vi "Aim Robot.vi"(10 "Drive Speed":dbl, 11 "RobotDriveDevRef":T1={"DevStatus"={"status"=FALSE, "code"=0, "source"=""}, "Motors[]"=[], "Square Inputs"=FALSE, "Max Output"=1.0}) -> (0 "Error Out":string, 3 "RobotDriveDevRef Out":T1={"DevStatus"={"status"=FALSE, "code"=0, "source"=""}, "Motors[]"=[], "Square Inputs"=FALSE, "Max Output"=1.0})   [LabVIEW 2016]
uses:
  <vilib>/Rock Robotics/WPI/RobotDrive/WPI_RobotDriveDevRef.ctl
  <vilib>/Rock Robotics/WPI/MotorControl/WPI_MotorControlDeviceRef.ctl
  <vilib>/Rock Robotics/WPI/MotorControl/WPI_MotorControlType.ctl
  <vilib>/Rock Robotics/SystemInterfaces/DIO/FPGA_DIOPWMChannel.ctl
  <vilib>/Rock Robotics/WPI/PWM/WPI_PWMDeadband.ctl
  <vilib>/Rock Robotics/WPI/Relay/WPI_RelayValue.ctl
  Robot Global Data.vi
  <vilib>/Rock Robotics/Network Tables/NT Read Boolean.vi
  <vilib>/Rock Robotics/WPI/RobotDrive/WPI_RobotDriveArcadeDrive_Standard(NoSaturation).vi
  <vilib>/Rock Robotics/Network Tables/NT Write Numeric Array.vi
  <vilib>/Rock Robotics/Network Tables/NT Read Number.vi
panel:
  out "Drive Motor Values":dbl[](array[numeric])
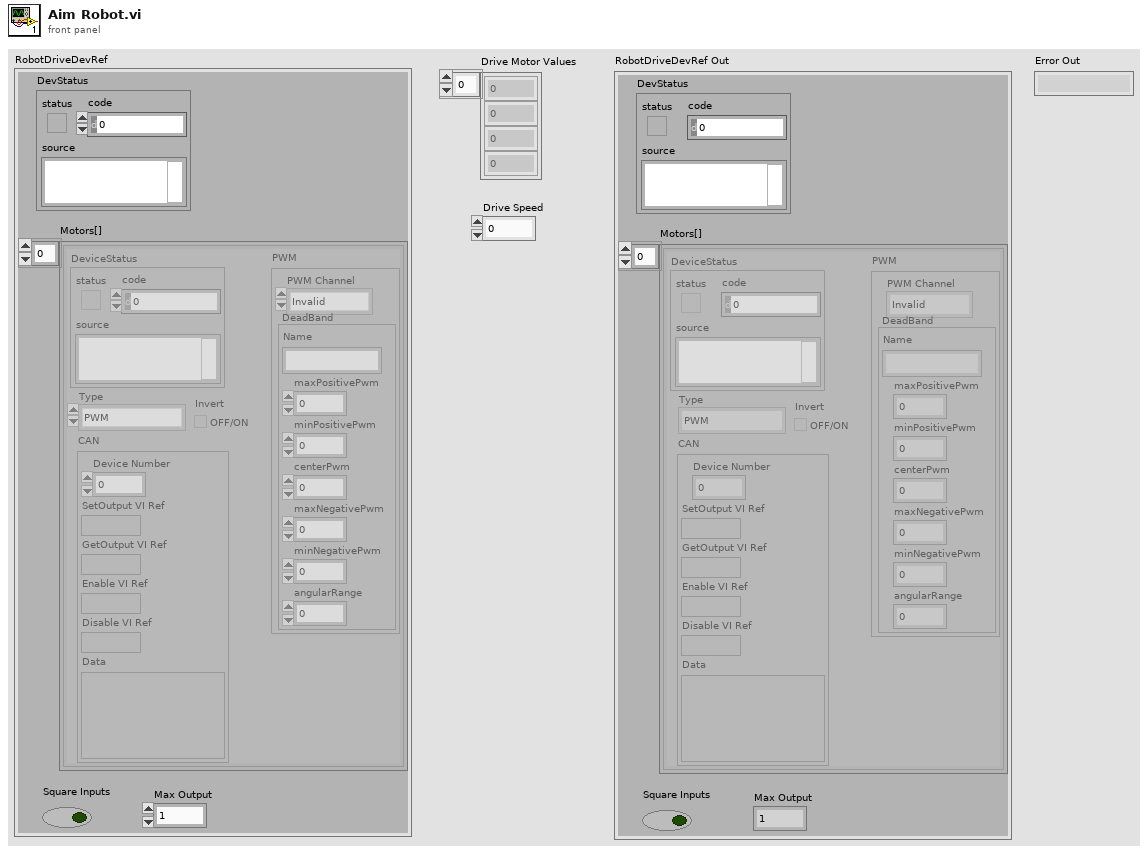
[diagram p1: front panel]
types:
  T1 = typedef "WPI_RobotDriveDevRef.ctl" = cluster{"DevStatus":errorcluster, "Motors[]":T2[], "Square Inputs":bool, "Max Output":dbl}
  T2 = typedef "WPI_MotorControlDeviceRef.ctl" = cluster{"DeviceStatus":errorcluster, "Type":T3, "PWM":cluster{"PWM Channel":T4, "DeadBand":T5}, "CAN":cluster{"Device Number":u8, "SetOutput VI Ref":variant, "GetOutput VI Ref":variant, "Enable VI Ref":variant, "Disable VI Ref":variant, "Data":variant}, "Invert":bool}
  T3 = typedef "WPI_MotorControlType.ctl" = enum16{"PWM", "CAN"}
  T4 = typedef "FPGA_DIOPWMChannel.ctl" = enum8{"PWM 0", "PWM 1", "PWM 2", "PWM 3", "PWM 4", "PWM 5", "PWM 6", "PWM 7", "PWM 8", "PWM 9", "PWM MXP 0", "PWM MXP 1", "PWM MXP 2", "PWM MXP 3", "PWM MXP 4", "PWM MXP 5", "PWM MXP 6", "PWM MXP 7", "PWM MXP 8", "PWM MXP 9", "Invalid"}
  T5 = typedef "WPI_PWMDeadband.ctl" = cluster{"Name":string, "maxPositivePwm":i32, "minPositivePwm":i32, "centerPwm":i32, "maxNegativePwm":i32, "minNegativePwm":i32, "angularRange":u16}
  T6 = typedef "WPI_RelayValue.ctl" = enum16{"Off", "On", "Forward", "Reverse"}
  T7 = typedef "WPI_RelayDevRef.ctl" = cluster{"DevStatus":errorcluster, "Relay Channel":T8, "Relay Direction":T9}
  T8 = typedef "FPGA_DIORelayChannel.ctl" = enum8{"Relay 0", "Relay 1", "Relay 2", "Relay 3", "Invalid"}
  T9 = typedef "WPI_RelayDirection.ctl" = enum16{"Both directions", "Forward only", "Reverse only"}
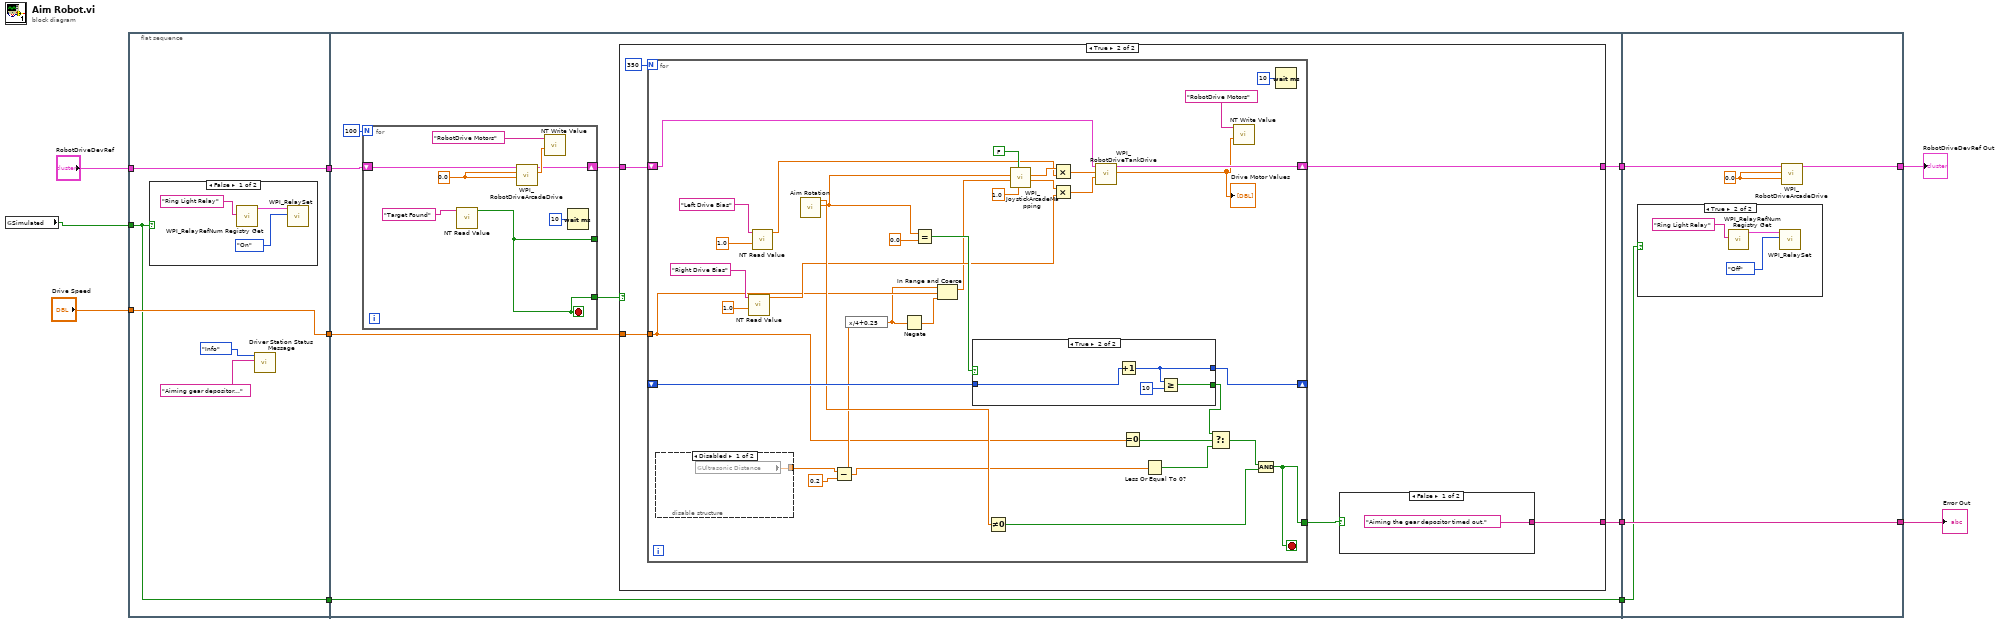
[diagram p0: block diagram]
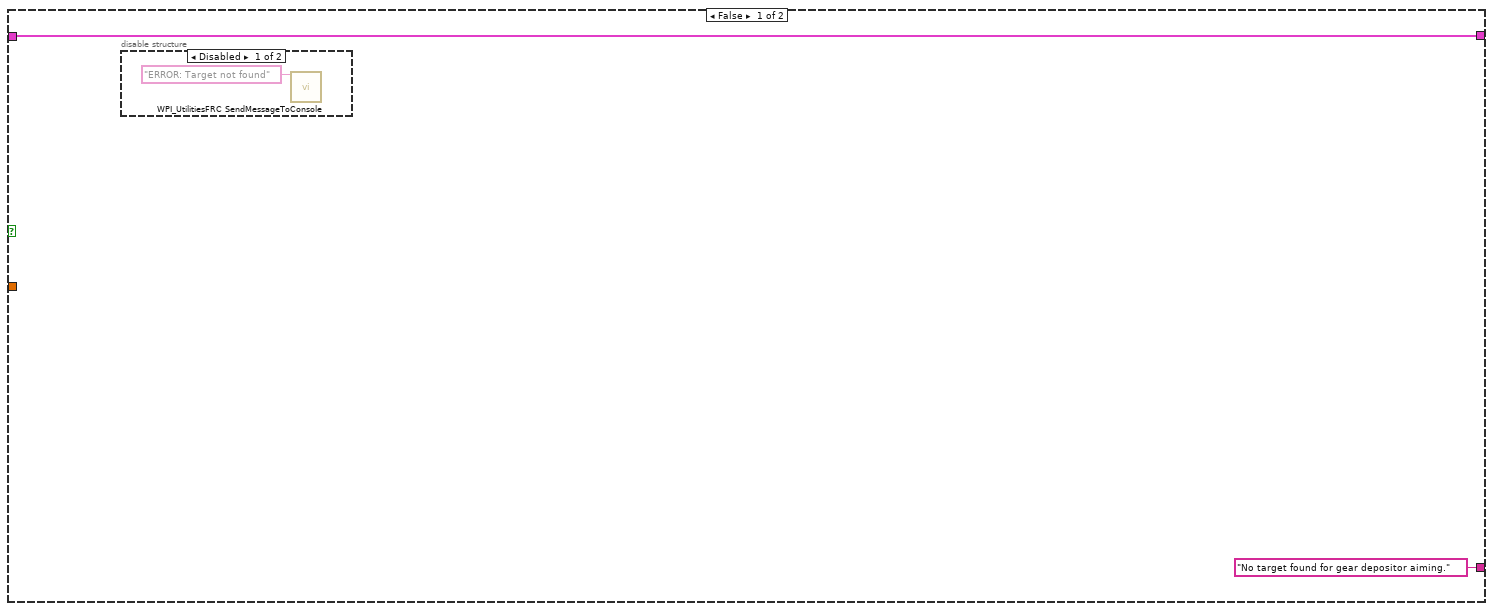
[diagram p3: hidden frame]
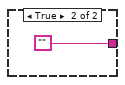
[diagram p5: hidden frame]
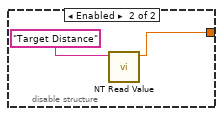
[diagram p6: hidden frame]
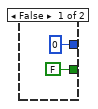
[diagram p7: hidden frame]
diagram:
  n1 = global read "Robot Global Data.vi" "Simulated"() -> (w3:bool)
  n2 = flat-sequence {
    tunnel: [w16] -> w11
    tunnel: "RobotDriveDevRef" -> [w16]
    tunnel: [w15] -> w9
    tunnel: "Drive Speed" -> [w15]
    tunnel: w3 -> [w12]
    tunnel: [w12] -> w1
    tunnel: w11 -> [w24]
    tunnel: w9 -> [w23]
    tunnel: [w22] -> w7
    tunnel: [w21] -> w5
    tunnel: [w20] -> w2
    tunnel: w1 -> [w20]
    tunnel: w7 -> [w96]
    tunnel: [w94] -> w6
    tunnel: w5 -> [w93]
    tunnel: [w93] -> w4
    tunnel: w2 -> [w92]
    frame #0 {
      n3 = case shown="False" w12 {
        frame False {
          n4 = call <vilib>:"WPI_RelayRefNum Registry Get.vi"("refnum name"="Ring Light Relay") -> ("RelayDevRef"=w18:T7)  [unwired: 9 in, 1 out]
          n5 = call <vilib>:"WPI_RelaySet.vi"("RelayValue"=WPI_RelayValue."On", "RelayDevRef"=w18) -> ()  [unwired: 8 in, 2 out]
        }
        frame True {
        }
      }
      n6 = call "Driver Station Status Message.vi"("Message"="Aiming gear depositor...", "Message Type"=enum16{"Error", "Warning", "Info"}."Info") -> ()  [unwired: 10 in]
    }
    frame #1 {
      n7 = for {
        N: 100 -> [_]
        tunnel: [w85] -> _
        shift-right: [w86] -> w26
        shift-left: w24 -> [w87]
        tunnel: [w85] -> w25
        stop <- w85 stop-if-true
        w84 = 0.0
        n8 = call-poly <vilib>:"NT Read Value.vi"("Name"="Target Found") -> ("Boolean"=w85:bool)  [unwired: 9 in, 1 out]
        n9 = call-poly <vilib>:"WPI_RobotDriveArcadeDrive.vi"("Y axis value"=w84, "X axis value"=w84, "RobotDriveDevRef"=w87) -> ("Motor Values"=w89:dbl[], "RobotDriveDevRef"=w86:T1)  [unwired: 6 in, 1 out]
        n10 = call-poly <vilib>:"NT Write Value.vi"("Numeric Array"=w89, "Name"="RobotDrive Motors") -> ()  [unwired: 9 in, 1 out]
        n11 = Wait (ms)(milliseconds to wait=u32 10) -> ()  [unwired: 1 out]
      }
      n12 = case shown="True" w25 {
        tunnel: w26 -> [w29 w35]
        tunnel: w23 -> [_ w34]
        tunnel: [w29 w33] -> w22
        tunnel: ["No target found for gear depositor aiming." w31] -> w21
        frame False {
          n13 = disable-structure shown="Disabled" {
            frame Disabled {
              n14 = call <vilib>:"WPI_UtilitiesFRC SendMessageToConsole.vi"("Message"="ERROR: Target not found") -> ()  [unwired: 14 in, 1 out]
            }
            frame Enabled {
            }
          }
        }
        frame True {
          n15 = for {
            N: 350 -> [_]
            shift-right: [w54] -> w33
            shift-left: w35 -> [w55]
            shift-right: [w71] -> _
            shift-left: _ -> [w72]
            tunnel: w34 -> [w42]
            tunnel: [w50] -> w32
            stop <- w50 stop-if-true
            n16 = disable-structure shown="Disabled" {
              disable-tunnel: [w75 w76] -> w44
              frame Disabled {
                n17 = global read "Robot Global Data.vi" "Ultrasonic Distance"() -> (w75:dbl)
              }
              frame Enabled {
                n18 = call-poly <vilib>:"NT Read Value.vi"("Name"="Target Distance") -> ("Numeric"=w76:dbl)  [unwired: 9 in, 1 out]
              }
            }
            n19 = call-poly <vilib>:"NT Read Value.vi"("Default Value"=1.0, "Name"="Right Drive Bias") -> ("Numeric"=w58:dbl)  [unwired: 8 in, 1 out]
            n20 = call-poly <vilib>:"NT Read Value.vi"("Default Value"=1.0, "Name"="Left Drive Bias") -> ("Numeric"=w59:dbl)  [unwired: 8 in, 1 out]
            n21 = call "Aim Rotation.vi"() -> ("Rotation"=w62:dbl, "Image Size X"=w68:dbl)  [unwired: 10 in]
            n22 = Subtract(x=w44, y=0.2) -> (x-y=w43:dbl)
            n23 = expression code="x/4+0.25"(w43) -> (w41:dbl)
            n24 = Negate(x=w41) -> (-x=w40:dbl)
            n25 = Equal?(x=w62, y=0.0) -> (x = y?=w69:bool)
            n26 = In Range and Coerce(upper limit=w41, x=w42, lower limit=w40) -> (coerced(x)=w39:dbl)  [unwired: 1 out]
            n27 = case shown="True" w69 {
              tunnel: [0 w82] -> w71
              tunnel: w72 -> [_ w83]
              tunnel: [FALSE w80] -> w48
              frame False {
              }
              frame True {
                n28 = Increment(x=w83) -> (x+1=w82:i32)
                n29 = Greater Or Equal?(x=w82, y=10) -> (x >= y?=w80:bool)
              }
            }
            n30 = Not Equal To 0?(x=w68) -> (x != 0?=w67:bool)
            n31 = call <vilib>:"WPI_JoystickArcadeMapping.vi"("Max Output"=1.0, "Square Inputs"=FALSE, "Y axis value"=w39, "X axis value"=w62) -> ("Right Motor Value"=w61:dbl, "Left Motor Value"=w60:dbl)  [unwired: 6 in]
            n32 = Multiply(x=w60, y=w59) -> (x*y=w57:dbl)
            n33 = Multiply(x=w61, y=w58) -> (x*y=w56:dbl)
            n34 = call <vilib>:"WPI_RobotDriveTankDrive.vi"("Right axis value"=w56, "Left axis value"=w57, "RobotDriveDevRef"=w55) -> ("Motor Values"=w53:dbl[], "RobotDriveDevRef"=w54:T1)  [unwired: 6 in, 1 out]
            "Drive Motor Values" <- w53
            n35 = Equal To 0?(x=w42) -> (x = 0?=w49:bool)
            n36 = Less Or Equal To 0?(x=w43) -> (x <= 0?=w47:bool)
            n37 = Select(t=w48, s=w49, f=w47) -> (s? t:f=w46:bool)
            n38 = call-poly <vilib>:"NT Write Value.vi"("Numeric Array"=w53, "Name"="RobotDrive Motors") -> ()  [unwired: 9 in, 1 out]
            n39 = Compound Arithmetic op=AND(w46, w67) -> (w50:bool)
            n40 = Wait (ms)(milliseconds to wait=u32 10) -> ()  [unwired: 1 out]
          }
          n41 = case shown="False" w32 {
            tunnel: ["Aiming the gear depositor timed out." ""] -> w31
            frame False {
            }
            frame True {
            }
          }
        }
      }
    }
    frame #2 {
      w95 = 0.0 ("X axis value")
      n42 = case shown="True" w92 {
        frame False {
        }
        frame True {
          n43 = call <vilib>:"WPI_RelayRefNum Registry Get.vi"("refnum name"="Ring Light Relay") -> ("RelayDevRef"=w98:T7)  [unwired: 9 in, 1 out]
          n44 = call <vilib>:"WPI_RelaySet.vi"("RelayValue"=WPI_RelayValue."Off", "RelayDevRef"=w98) -> ()  [unwired: 8 in, 2 out]
        }
      }
      n45 = call-poly <vilib>:"WPI_RobotDriveArcadeDrive.vi"("Y axis value"=w95, "X axis value"=w95, "RobotDriveDevRef"=w96) -> ("RobotDriveDevRef"=w94:T1)  [unwired: 6 in, 2 out]
    }
  }
  "RobotDriveDevRef Out" <- w6
  "Error Out" <- w4
